vi "SigGen_ESG_MatchIDNStr.vi"(8 "error in":errorcluster, 10 "IDNStr":string) -> (0 "error out":errorcluster, 2 "IDN match":bool, 3 "ClassLibraryFile":path)   [LabVIEW 2014]
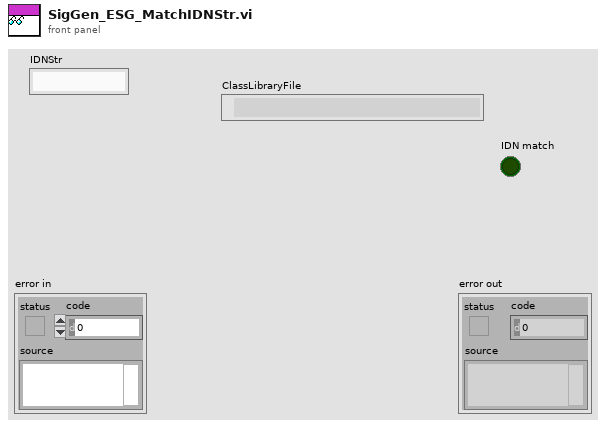
[diagram p1: front panel]
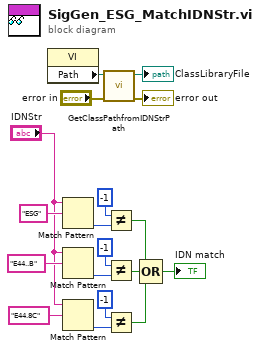
[diagram p0: block diagram]
diagram:
  n1 = property class="VI"() -> ("Path"=w18:path)  [unwired: 2 in, 2 out]
  n2 = Match Pattern(string="IDNStr", regular expression="ESG") -> (offset past match=w7:i32)  [unwired: 1 in, 3 out]
  n3 = Match Pattern(string="IDNStr", regular expression="E44..B") -> (offset past match=w12:i32)  [unwired: 1 in, 3 out]
  n4 = Match Pattern(string="IDNStr", regular expression="E44.8C") -> (offset past match=w13:i32)  [unwired: 1 in, 3 out]
  n5 = call "GetClassPathfromIDNStrPath.vi"("error in (no error)"="error in", "Path in"=w18) -> ("error out"=→"error out":errorcluster, "Path out"=→"ClassLibraryFile":path)  [unwired: 8 in]
  n6 = Not Equal?(x=-1, y=w7) -> (x != y?=w4:bool)
  n7 = Not Equal?(x=-1, y=w12) -> (x != y?=w5:bool)
  n8 = Not Equal?(x=-1, y=w13) -> (x != y?=w3:bool)
  n9 = Compound Arithmetic op=OR(w4, w5, w3) -> (→"IDN match":bool)
